vi "get controller information.vi"(10 "Device Model":enum16{"cRIO-9068"}(ring)) -> (0 "error out":errorcluster, 2 "passed?":bool)   [LabVIEW 2016, in "SMI Tests.lvlib"]
uses:
  SMI Tests.lvlib
  classes/SysCfg Device/SysCfg Device.lvclass
  classes/Controller/Controller.lvclass
  <vilib>/utf/common/utf_test_result.ctl
  <vilib>/utf/NI_UnitTestFramework.lvlib
  <vilib>/utf/common/utf_vi_tag.ctl
  <vilib>/utf/common/utf_test_comparison_operators.ctl
  <vilib>/utf/common/utf_test_result_failure.ctl
  <vilib>/utf/common/utf_test_result_troll.ctl
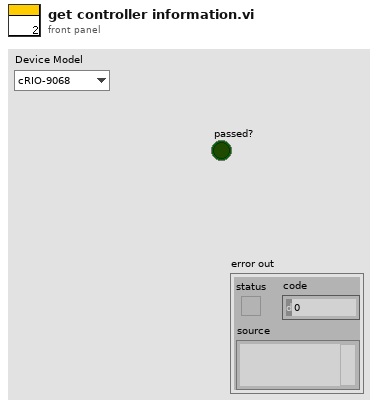
[diagram p1: front panel]
types:
  T1 = typedef "SMI.lvlib/Controller.lvclass/ControllerInformation.ctl" = cluster{"SysCfg Session":refnum<data-value>, "System Hardware Reference":refnum<data-value>, "Vendor Name":string, "Product Name":string, "Product ID":u16, "Serial Number":string, "Device Information":T2, "Primary Network Adapter":T3, "Secondary Network Adapters":T3[]}
  T2 = typedef "SMI.lvlib/Controller.lvclass/DeviceInformation.ctl" = cluster{"Resource":string, "Device Class":string, "System Start Time":timestamp, "Current Time":timestamp, "Time Zone":string, "Firmware Revision":string, "Image Title":string, "Image Version":string, "System Status":string}
  T3 = typedef "SMI.lvlib/Controller.lvclass/NetworkAdapterSettings.ctl" = cluster{"IP Address":string, "MAC Address":string, "IP Address Request Mode":u32, "SubnetMask":string, "Gateway":string, "DNS Server":string, "Adapter Mode":u32, "Adapter Type":u32}
  T4 = typedef "NI_UnitTestFramework.lvlib/utf_test_result_troll.ctl" = cluster{"time elapsed [ms]":u32, "result (test)":T5, "result (parameters)":T6[]}
  T5 = typedef "NI_UnitTestFramework.lvlib/utf_test_result.ctl" = enum16{"Passed", "Failed", "Error", "Skipped", "Not Processed"}
  T6 = typedef "NI_UnitTestFramework.lvlib/utf_test_result_failure.ctl" = cluster{"result":T5, "error message":string, "parameter name":string, "parameter value":variant, "parameters":variant[], "comparison":T7, "requirement ID":string, "VI":T8, "Used Vector Name":string}
  T7 = typedef "NI_UnitTestFramework.lvlib/utf_test_comparison_operators.ctl" = enum16{"=", "!=", ">", ">=", "<", "<=", "range", "symmetric tolerance", "asymmetric tolerance", "string contains", "string not contain", "array size", "string length", "array range", "by element", "array range (limit array)", "user-defined", "array contains", "array not contain", "vector length", "= (elm)", "!= (elm)", "= (case insensitive)", "!= (case insensitive)"}
  T8 = typedef "NI_UnitTestFramework.lvlib/utf_vi_tag.ctl" = enum16{"Setup VI", "VI under Test", "Teardown VI"}
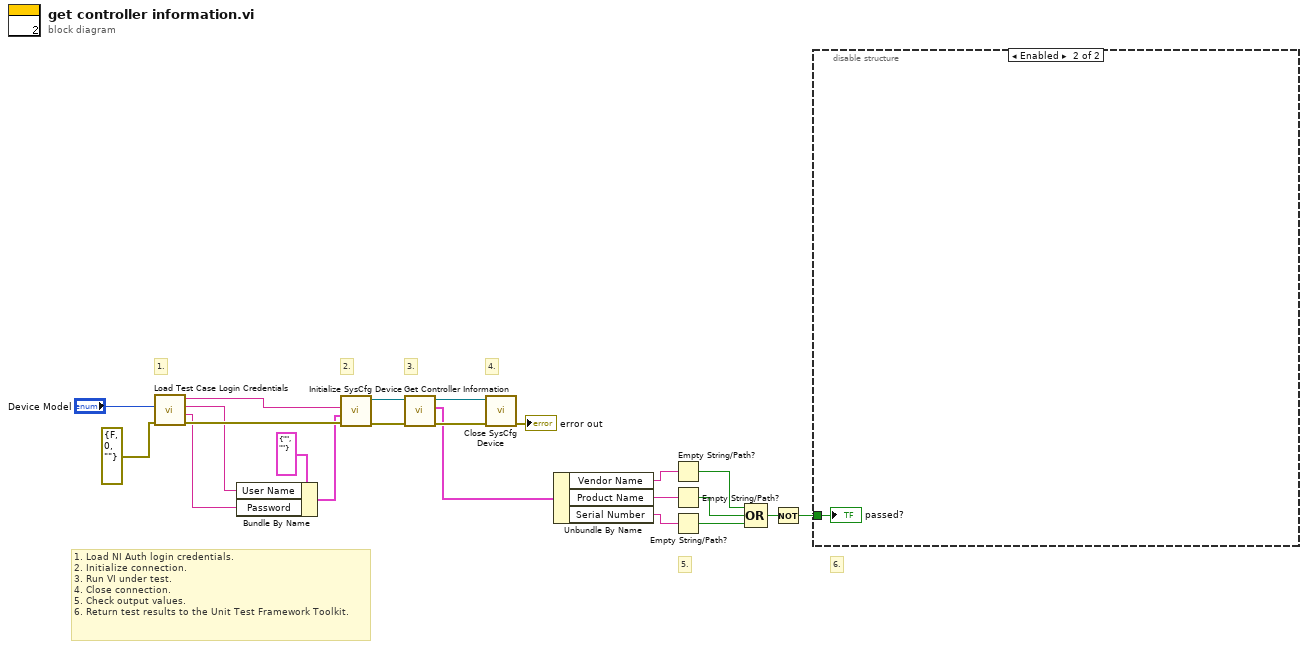
[diagram p0: block diagram]
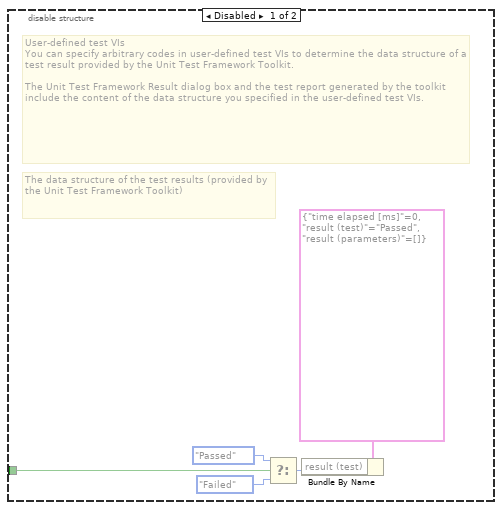
[diagram p2: hidden frame]
diagram:
  # "6."
  # "4."
  # "1. Load NI Auth login credentials.\n2. Initialize connection.\n3. Run VI under test.\n4. Close connection.\n5. Check output values.\n6. Return test results to the Unit Test Framework Toolkit."
  # "2."
  # "1."
  # "3."
  # "5."
  n1 = call "Load Test Case Login Credentials.vi"("error in"=errorcluster {"status"=FALSE, "code"=0, "source"=""}, "Device Model"="Device Model") -> ("error out"=w22:errorcluster, "Password"=w17:string, "Username"=w18:string, "IP Address"=w16:string)  [unwired: 6 in]
  n2 = Bundle By Name(cluster=cluster{"User Name":string, "Password":string} {"User Name"="", "Password"=""} ("NI Auth (Unconfigured)"), "User Name"=w18, "Password"=w17) -> (w15:cluster{"User Name":string, "Password":string})
  n3 = call "Initialize SysCfg Device.vi"("error in"=w22, "login"=w15, "target address (localhost)"=w16) -> ("error out"=w21:errorcluster, "Controller out"=w14:refnum<class "Controller.lvclass">)  [unwired: 7 in]
  n4 = call "Get Controller Information.vi"("error in"=w21, "Controller in"=w14) -> ("error out"=w20:errorcluster, "device information"=w11:T1, "Controller out"=w13:refnum<class "Controller.lvclass">)  [unwired: 7 in]
  n5 = call "Close SysCfg Device.vi"("error in"=w20, "Controller in"=w13) -> ("error out"=→"error out":errorcluster)  [unwired: 9 in]
  n6 = Unbundle By Name(w11) -> ("Vendor Name"=w8:string, "Product Name"=w7:string, "Serial Number"=w10:string)
  n7 = Empty String/Path?(string/path=w8) -> (empty?=w6:bool)
  n8 = Empty String/Path?(string/path=w7) -> (empty?=w5:bool)
  n9 = Empty String/Path?(string/path=w10) -> (empty?=w4:bool)
  n10 = Compound Arithmetic op=OR(w6, w5, w4) -> (w3:bool)
  n11 = Not(x=w3) -> (.not. x?=w2:bool)
  n12 = disable-structure shown="Enabled" {
    disable-tunnel: w2 -> [w23 w28]
    frame Disabled {
      # "User-defined test VIs\nYou can specify arbitrary codes in user-defined test VIs to determine the data structure of a test result provided by the Unit Test Framework Toolkit.\n\nThe Unit Test Framework Result dialog box and the test report generated by the toolkit include the content of the data structure you specified in the user-defined test VIs."
      # "The data structure of the test results (provided by the Unit Test Framework Toolkit)"
      n13 = Select(t=utf_test_result."Passed" ("Result (Test)"), s=w23, f=utf_test_result."Failed" ("Result (Test)")) -> (s? t:f=w27:T5)
      n14 = Bundle By Name(cluster=T4 {"time elapsed [ms]"=0, "result (test)"=enum."Passed", "result (parameters)"=[]} ("Constant"), "result (test)"=w27) -> ()  [unwired: 1 out]
    }
    frame Enabled {
      "passed?" <- w28
    }
  }
